vi "Arrange Node.vi"(8 "error in (no error)":errorcluster, 10 "Arrange":T1, 11 "Node in":refnum<vi>) -> (0 "error out":errorcluster, 3 "Node out":refnum<vi>)   [LabVIEW 2019, in "Builtins.lvlib"]
doc: "Arrange node terminal positions and adjust for custom terminal offsets.\n\nCreated by: Ryan Pacini"
uses:
  Builtins.lvlib
  Arrange.ctl
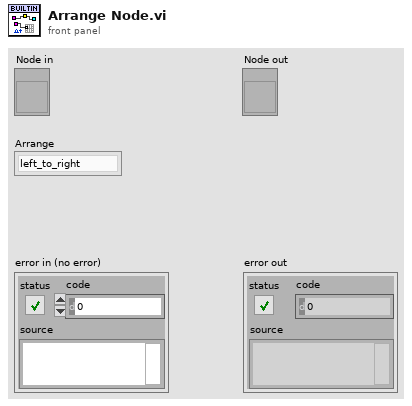
[diagram p1: front panel]
types:
  T1 = typedef "Builtins.lvlib/Arrange.ctl" = enum8{"left_to_right", "right_to_left"}
  T2 = cluster{"Position":cluster{"h":i16, "v":i16}, "Flags":i32, "Type":enum32{"LooseEnd", "Endpoint", "Bend", "Junction"}, "Up Joint Index":i16, "Down Joint Index":i16, "Left Joint Index":i16, "Right Joint Index":i16}[]
  T3 = typedef "LVRectTypeDef.ctl" = cluster{"Left":i16, "Top":i16, "Right":i16, "Bottom":i16}
  T4 = typedef "LVPositionTypeDef.ctl" = cluster{"Left":i32, "Top":i32}
  T5 = cluster{"Left":i32, "Top":i32, "Right":i32, "Bottom":i32}
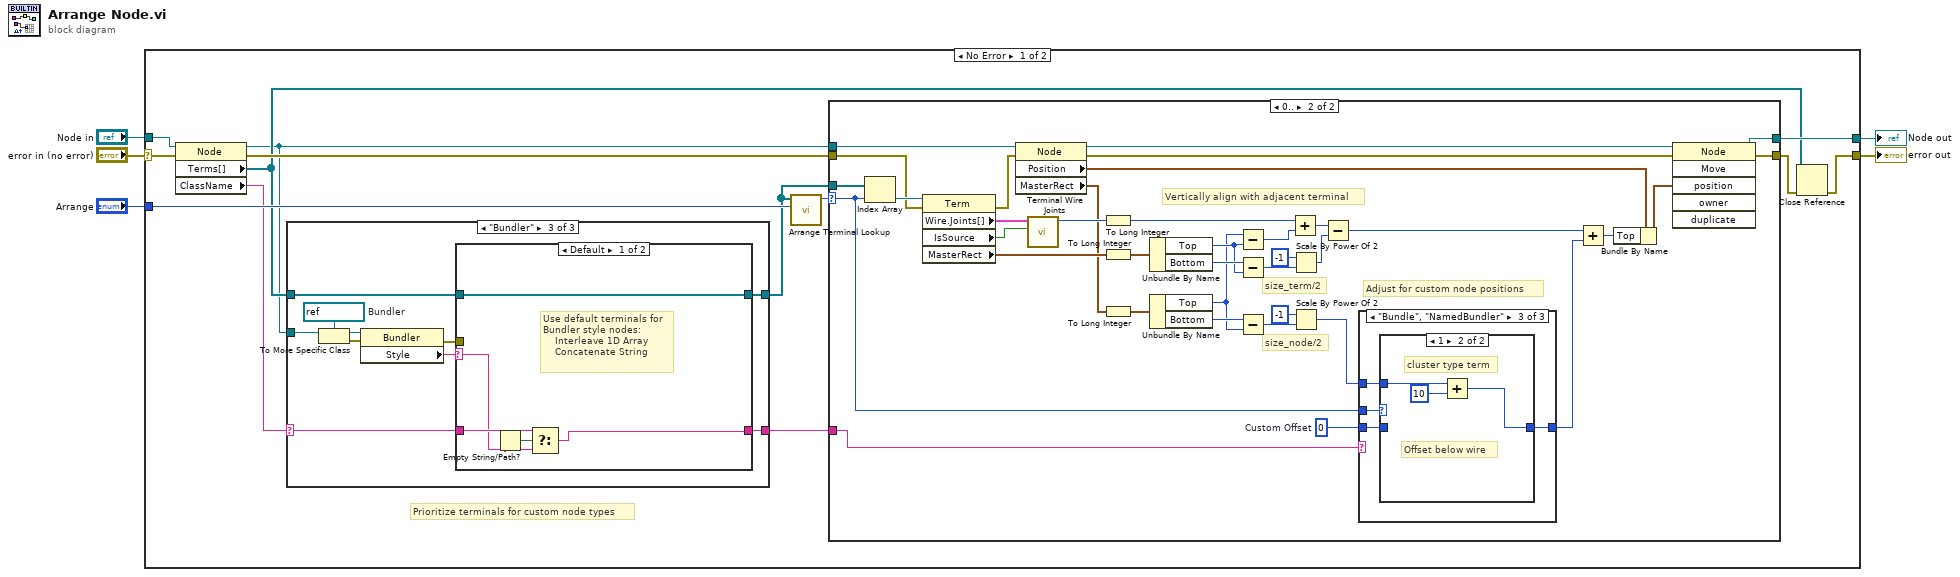
[diagram p0: block diagram]
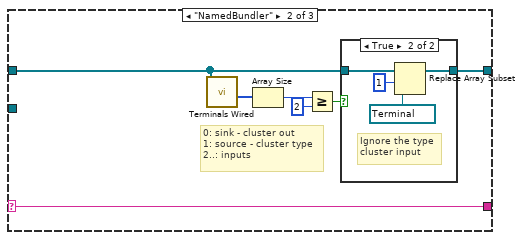
[diagram p3: hidden frame]
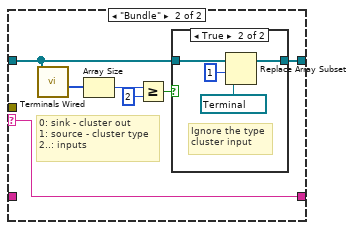
[diagram p5: hidden frame]
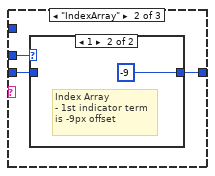
[diagram p9: hidden frame]
diagram:
  n1 = case shown="No Error" "error in (no error)" {
    selector: "error in (no error)" -> [w14 w113]
    tunnel: "Arrange" -> [w15 _]
    tunnel: "Node in" -> [w13 w114]
    tunnel: [w12 w113] -> w2
    tunnel: [w11 w114] -> w1
    frame No Error {
      # "Prioritize terminals for custom node types"
      n2 = property class="Node"(reference=w13, error in=w14) -> (reference out=w7:refnum<vi>, error out=w18:errorcluster, "Terms[]"=w10:refnum<vi>[], "ClassName"=w6:string)
      n3 = case shown="\"Bundler\"" w6 {
        selector: w6 -> [w19 w21 w35]
        tunnel: w10 -> [w20 w26 w41]
        tunnel: [w20 w27 w42] -> w9
        tunnel: [w19 w21 w36] -> w8
        tunnel: w7 -> [_ _ w40]
        frame Default {
        }
        frame "NamedBundler" {
          # "0: sink - cluster out\n1: source - cluster type\n2..: inputs"
          n4 = call "Terminals Wired.vi"("Terminals"=w26) -> ("Node Input indexes"=w24:i32[])  [unwired: 8 in, 2 out]
          n5 = Array Size(array=w24) -> (size(s)=w22:i32)
          n6 = Greater Or Equal?(x=w22, y=2) -> (x >= y?=w23:bool)
          n7 = case shown="True" w23 {
            tunnel: [w28 w32] -> w27
            tunnel: w26 -> [w28 w31]
            frame False {
            }
            frame True {
              # "Ignore the type\ncluster input"
              n8 = Replace Array Subset(array=w31, new element=refnum<vi> refnum ("new element/subarray"), index=1) -> (w32:refnum<vi>[])
            }
          }
        }
        frame "Bundler" {
          w39 = refnum<vi> refnum  # Bundler
          n9 = To More Specific Class(target class=w39, reference=w40) -> (specific class reference=w38:refnum<vi>, error out=w37:errorcluster)  [unwired: 1 in]
          n10 = property class="Bundler"(reference=w38, error in=w37) -> (error out=w33:errorcluster, "Style"=w34:string)  [unwired: 1 out]
          n11 = case shown="Default" w34 {
            selector: w34 -> [w44 w48]
            tunnel: [w47 w54] -> w42
            tunnel: w41 -> [w47 w53]
            tunnel: [w43 w48] -> w36
            tunnel: w35 -> [w45 _]
            tunnel: w33 -> [_ _]
            frame Default {
              # "Use default terminals for\nBundler style nodes:\n    Interleave 1D Array\n    Concatenate String"
              n12 = Empty String/Path?(string/path=w44) -> (empty?=w46:bool)
              n13 = Select(t=w45, s=w46, f=w44) -> (s? t:f=w43:string)
            }
            frame "Bundle" {
              # "0: sink - cluster out\n1: source - cluster type\n2..: inputs"
              n14 = call "Terminals Wired.vi"("Terminals"=w53) -> ("Node Input indexes"=w51:i32[])  [unwired: 8 in, 2 out]
              n15 = Array Size(array=w51) -> (size(s)=w49:i32)
              n16 = Greater Or Equal?(x=w49, y=2) -> (x >= y?=w50:bool)
              n17 = case shown="True" w50 {
                tunnel: [w55 w59] -> w54
                tunnel: w53 -> [w55 w58]
                frame False {
                }
                frame True {
                  # "Ignore the type\ncluster input"
                  n18 = Replace Array Subset(array=w58, new element=refnum<vi> refnum ("new element/subarray"), index=1) -> (w59:refnum<vi>[])
                }
              }
            }
          }
        }
      }
      n19 = call "Arrange Terminal Lookup.vi"("Arrange"=w15, "Terminals"=w9) -> ("Terminal Index"=w17:i32)  [unwired: 9 in]
      n20 = case shown="0.." w17 {
        selector: w17 -> [_ w76]
        tunnel: [w61 w98] -> w16
        tunnel: w7 -> [w60 w93]
        tunnel: w18 -> [w61 w88]
        tunnel: w9 -> [_ w72]
        tunnel: w8 -> [_ w75]
        tunnel: [w60 w73] -> w11
        frame ..-1 {
        }
        frame 0.. {
          w78 = 0  # Custom Offset
          # "Adjust for custom node positions"
          # "size_node/2"
          # "size_term/2"
          # "Vertically align with adjacent terminal"
          n21 = Index Array(array=w72, index=w76) -> (element=w90:refnum<vi>)
          n22 = property class="Term"(reference=w90, error in=w88) -> (error out=w89:errorcluster, "Wire.Joints[]"=w91:T2, "IsSource"=w74:bool, "MasterRect"=w87:T3)  [unwired: 1 out]
          n23 = property class="Node"(reference=w93, error in=w89) -> (reference out=w96:refnum<vi>, error out=w97:errorcluster, "Position"=w95:T4, "MasterRect"=w71:T3)
          n24 = call "Terminal Wire Joints.vi"("Is Source?"=w74, "Joints"=w91) -> ("Vertical Position"=w92:i16)  [unwired: 8 in, 1 out]
          n25 = To Long Integer(number=w92) -> (32bit integer=w85:i32)
          n26 = To Long Integer(number=w87) -> (32bit integer=w83:T5)
          n27 = To Long Integer(number=w71) -> (32bit integer=w69:T5)
          n28 = Unbundle By Name(w83) -> ("Top"=w82:i32, "Bottom"=w86:i32)
          n29 = Unbundle By Name(w69) -> ("Top"=w68:i32, "Bottom"=w70:i32)
          n30 = Subtract(x=w68, y=w82) -> (x-y=w84:i32)
          n31 = Subtract(x=w86, y=w82) -> (x-y=w64:i32)
          n32 = Subtract(x=w70, y=w68) -> (x-y=w67:i32)
          n33 = Add(x=w85, y=w84) -> (x+y=w81:i32)
          n34 = Scale By Power Of 2(n=i16 -1, x=w64) -> (x*2^n=w63:i32)
          n35 = Scale By Power Of 2(n=i16 -1, x=w67) -> (x*2^n=w62:i32)
          n36 = Subtract(x=w81, y=w63) -> (x-y=w80:i32)
          n37 = case shown="\"Bundle\", \"NamedBundler\"" w75 {
            tunnel: w76 -> [_ w102 w108]
            tunnel: [w99 w101 w107] -> w77
            tunnel: w78 -> [w99 w100 w106]
            tunnel: w62 -> [_ _ w105]
            frame Default {
            }
            frame "IndexArray" {
              n38 = case shown="1" w102 {
                tunnel: [w103 -9 ("Vertical Offset")] -> w101
                tunnel: w100 -> [w103 _]
                frame Default {
                }
                frame 1 {
                  # "Index Array\n- 1st indicator term\nis -9px offset"
                }
              }
            }
            frame "Bundle", "NamedBundler" {
              n39 = case shown="1" w108 {
                tunnel: [w109 w110] -> w107
                tunnel: w106 -> [w109 _]
                tunnel: w105 -> [_ w112]
                frame Default {
                }
                frame 1 {
                  # "cluster type term"
                  # "Offset below wire"
                  n40 = Add(x=w112, y=10 ("Vertical Offset")) -> (x+y=w110:i32)
                }
              }
            }
          }
          n41 = Add(x=w80, y=w77) -> (x+y=w79:i32)
          n42 = Bundle By Name(cluster=w95, "Top"=w79) -> (w94:T4)
          n43 = invoke class="Node" method="Move"(reference=w96, error in=w97, "position"=w94) -> (reference out=w73:refnum<vi>, error out=w98:errorcluster)  [unwired: 3 in, 4 out]
        }
      }
      n44 = Close Reference(reference=w10, error in (no error)=w16) -> (error out=w12:errorcluster)
    }
    frame Error {
    }
  }
  "error out" <- w2
  "Node out" <- w1
